vi "run_cursor.vi"(6 "ms timeout (0:default)":i32, 8 "error in (no error)":errorcluster, 10 "query":string, 11 "rethinkdb in":T2) -> (0 "error out":errorcluster, 2 "cursor":T1, 3 "rethinkdb out":T2)   [LabVIEW 2017, in "rethinkdb.lvlib"]
uses:
  rethinkdb.lvlib
  refnum.ctl
  cursor_refnum.ctl
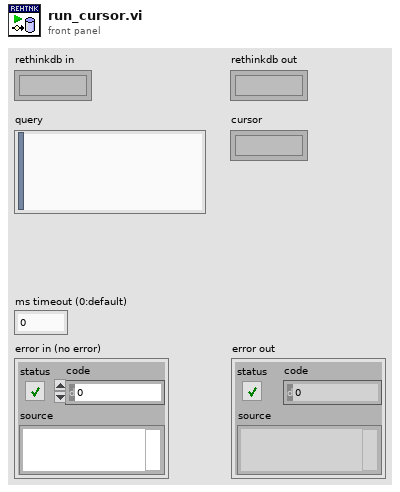
[diagram p1: front panel]
types:
  T1 = typedef "rethinkdb.lvlib/cursor_refnum.ctl" = refnum<k1>
  T2 = typedef "rethinkdb.lvlib/refnum.ctl" = refnum<k1>
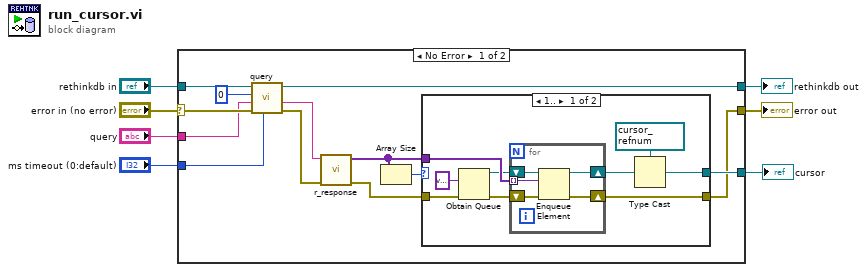
[diagram p0: block diagram]
diagram:
  n1 = case shown="No Error" "error in (no error)" {
    selector: "error in (no error)" -> [w20 w37]
    tunnel: "ms timeout (0:default)" -> [w19 _]
    tunnel: "query" -> [w18 _]
    tunnel: "rethinkdb in" -> [w17 w36]
    tunnel: [w16 w36] -> w3
    tunnel: [w9 w37] -> w2
    tunnel: [w10 _] -> w1
    frame No Error {
      n2 = call "query.vi"("ms timeout (0:default)"=w19, "error in (no error)"=w20, "query"=w18, "token in (random)"=u64 0, "rethinkdb in"=w17) -> ("error out"=w13:errorcluster, "response"=w14:string, "rethinkdb out"=w16:T2)  [unwired: 3 in, 1 out]
      n3 = call "r_response.vi"("error in (no error)"=w13, "response"=w14) -> ("error out"=w8:errorcluster, "values"=w12:variant[])  [unwired: 8 in]
      n4 = Array Size(array=w12) -> (size(s)=w11:i32)
      n5 = case shown="1.." w11 {
        tunnel: w12 -> [w27 _]
        tunnel: [w22 _] -> w10
        tunnel: w8 -> [w24 w35]
        tunnel: [w28 w35] -> w9
        frame 1.. {
          w21 = T1 refnum items=["cursor"] ("cursor 2")
          n6 = Obtain Queue(element data type=variant, error in (no error)=w24) -> (queue out=w23:refnum<queue>, error out=w25:errorcluster)  [unwired: 3 in, 1 out]
          n7 = for {
            tunnel: w27 -> [w30] mode=indexing
            shift-right: [w31] -> w28
            shift-left: w25 -> [w34]
            shift-right: [w32] -> w29
            shift-left: w23 -> [w33]
            n8 = Enqueue Element(queue=w33, element=w30, error in (no error)=w34) -> (queue out=w32:refnum<queue>, error out=w31:errorcluster)  [unwired: 1 in, 1 out]
          }
          n9 = Type Cast(type=w21, x=w29) -> (*(type *) &x=w22:T1)
        }
        frame ..0 {
        }
      }
    }
    frame Error {
    }
  }
  "error out" <- w2
  "rethinkdb out" <- w3
  "cursor" <- w1
